vi "PH_PPPA_PowerUnit.PC_StateDumpRoss.vi"(0 "i ref in":refnum<vi>, 3 "Dump Ross State":T1 items=["no info", "off/false/out", "on/true/in", "Failure", "Alarm", "Status 1", "Status 2", "Status 3"], 4 "not linked":bool, 5 "error in (no error)":errorcluster) -> (14 "i ref out":refnum<vi>, 19 "error out":errorcluster)   [LabVIEW 2014, in "PH_PPPA_PowerUnit.lvlib"]
doc: "This VI writes the Dump Ross Relais Tag values to own attributes, calculates the state of the device and sets the GUI object."
uses:
  PH_PPPA_PowerUnit.lvlib
  PH_StatusHandler/PH_StatusHandler.Status.ctl
  PH_Common/PH_Common.lvlib
  PH_StatusHandler/PH_StatusHandler.lvlib
  PH_Beckhoff_PP_PU/PH_Beckhoff_PP_PU.lvlib
  PH_PowerUnit_BaseClass/PH_PowerUnit_BaseClass.lvlib
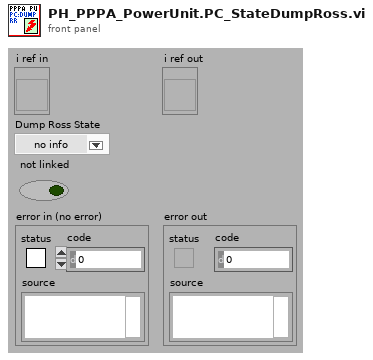
[diagram p1: front panel]
types:
  T1 = typedef "PH_StatusHandler.lvlib/PH_StatusHandler.Status.ctl" = i16
  T2 = typedef "PH_PowerUnit_BaseClass.lvlib/PH_PowerUnit_BaseClass.i attribute.ctl" = cluster{"Constructor finished":bool, "PU":cluster{"In use":bool, "Service ID in use":i32, "GUI Ref":refnum<vi>}, "Enabling":cluster{"State":T3, "GUI Ref":refnum<vi>}, "Timing":cluster{"Last Shot":dbl, "Time between Shots [Sec]":dbl, "Waiting Time over?":bool, "Service ID Waiting Time":i32, "GUI Ref":refnum<vi>, "Instance":cluster{"Status":T1, "linked?":bool, "GUI Ref":refnum<vi>}}, "Sequencer":cluster{"SM State":string, "GUI Ref":refnum<vi>, "linked":bool}, "Subscribed Trendmssgs":cluster{"Tagname":string, "Status":T1, "linked?":bool, "Shot Condition":T1, "GUI Ref":refnum<vi>}[], "PP PU":T4, "Default Voltage (V)":dbl, "GUI Refs":T5, "PSDB data":cluster{"Shot Voltage [V]":dbl, "State TO SM":T6, "Write 2 early":bool}, "State TO SM":T6}
  T3 = typedef "PH_SystemInformation.lvlib/PH_SystemInformationEnabling State.ctl" = i32
  T4 = typedef "PH_PP_Common.lvlib/PH_PP_Common.PUs.ctl" = enum16{"no Info", "PA-19mm-1", "PA-19mm-2", "PA-45mm-PILC", "PA-45mm-MAIN", "MA-PU-1", "MA-PU-2", "MA-PU-3", "MA-PU-4", "MA-PU-5", "MA-PU-6", "MA-FR", "MA-PILC", "PA-45mm-DP"}
  T5 = typedef "PH_PowerUnit_BaseClass.lvlib/PH_PowerUnit_BaseClass.GUI Refs.ctl" = cluster{"Delete Inst":refnum<vi>, "State TO SM":refnum<vi>, "State SM":refnum<vi>, "Fire":refnum<vi>}
  T6 = typedef "PH_PowerUnit_BaseClass.lvlib/PH_PowerUnit_BaseClass.SM States.ctl" = enum16{".", "Stand by", "Switch PU on", "Configure", "Set Default Voltage", "Set STANDBY", "Set READY", "Wait for Shot Cmd", "Open Dump Rods", "Open Ross Relais", "Close Ross Relais", "Switch PSU on", "Switch PSU off", "Charge", "Switch GD Channel on", "Close Dump Rods", "Rods-TO", "RR-TO", "PSU-TO", "Trigger-TO"}
  T7 = typedef "PH_PPPA_PowerUnit.lvlib/PH_PPPA_PowerUnit.i attribute.ctl" = cluster{"GUI Refs":cluster{"Ignitron":refnum<vi>, "Rossrelais":refnum<vi>, "Set Voltage":refnum<vi>, "PSU":refnum<vi>, "EOC":refnum<vi>, "Trigger":refnum<vi>}, "Ignitron":T8, "PSU":T9, "Dump Ross Relais":T10, "Trigger":cluster{"State Device":T1, "linked?":bool}, "Timing Settings":cluster{"Prdc Fast?":bool, "Default Value Periodic Interval":i32, "Mercury on since":dbl, "Warm up Time Mercury [s]":dbl}, "Set Voltage [V]":dbl, "19er Ignitionbox":string}
  T8 = typedef "PH_PP_Common.lvlib/PH_PP_Common.Ignitron Attributes.ctl" = cluster{"State Device":T1, "linked?":bool}
  T9 = typedef "PH_PP_Common.lvlib/PH_PP_Common.PSU Attributes.ctl" = cluster{"lower limit [V]":dbl, "upper limit [V]":dbl, "Voltage set":bool, "State Device":T1, "linked?":bool}
  T10 = typedef "PH_PP_Common.lvlib/PH_PP_Common.Ross Relais Attributes.ctl" = cluster{"State Device":T1, "linked?":bool}
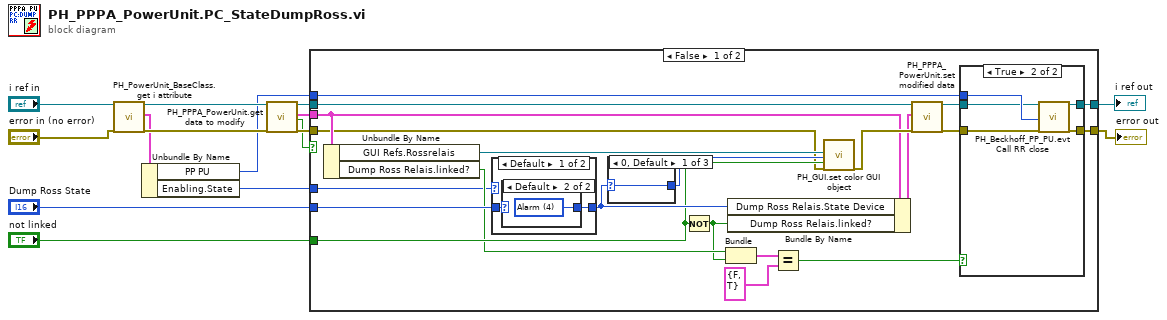
[diagram p0: block diagram]
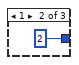
[diagram p3: hidden frame]
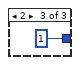
[diagram p4: hidden frame]
diagram:
  n1 = call "PH_PowerUnit_BaseClass.get i attribute.vi"("i ref in"="i ref in", "error in (no error)"="error in (no error)") -> ("i ref out"=w4:refnum<vi>, "i attribute"=w3:T2, "error out"=w6:errorcluster)  [unwired: 15 in]
  n2 = Unbundle By Name(w3) -> ("PP PU"=w1:T4, "Enabling.State"=w2:T3)
  n3 = call "PH_PPPA_PowerUnit.get data to modify.vi"("i ref in"=w4, "error in (no error)"=w6) -> ("i ref out"=w15:refnum<vi>, "i attribute"=w13:T7, "timed out"=w12:bool, "error out"=w14:errorcluster)  [unwired: 14 in]
  n4 = case shown="False" w12 {
    tunnel: w15 -> [w19 w53]
    tunnel: [w23 w53] -> w11
    tunnel: w14 -> [w18 w52]
    tunnel: [w21 w52] -> w10
    tunnel: w13 -> [w33 _]
    tunnel: "Dump Ross State" -> [w32 _]
    tunnel: "not linked" -> [w29 _]
    tunnel: w2 -> [w17 _]
    tunnel: w1 -> [w16 _]
    frame False {
      n5 = Unbundle By Name(w33) -> ("GUI Refs.Rossrelais"=w34:refnum<vi>, "Dump Ross Relais.linked?"=w28:bool)
      n6 = case shown="Default" w17 {
        tunnel: w32 -> [w48 w51]
        tunnel: [w47 w51] -> w31
        frame Default {
          n7 = case shown="Default" w48 {
            selector: w48 -> [w49 _]
            tunnel: [w49 w50] -> w47
            frame 2 {
            }
            frame Default {
              w50 = T1 4 items=["no info", "off/false/out", "on/true/in", "Failure", "Alarm", "Status 1", "Status 2", "Status 3"] ("Dump Ross State")
            }
          }
        }
        frame 1 {
        }
      }
      n8 = case shown="0, Default" w31 {
        selector: w31 -> [w44 _ _]
        tunnel: [w44 2 ("State") 1 ("State")] -> w30
        frame 0, Default {
        }
        frame 1 {
        }
        frame 2 {
        }
      }
      n9 = Not(x=w29) -> (.not. x?=w27:bool)
      n10 = Bundle("linked?"=w28, w27) -> (w26:cluster{"linked?":bool, bool})  [unwired: 1 in]
      n11 = Bundle By Name(cluster=w33, "Dump Ross Relais.State Device"=w31, "Dump Ross Relais.linked?"=w27) -> (w35:T7)
      n12 = Equal?(x=w26, y=cluster{"linked?":bool, bool} {"linked?"=FALSE, TRUE}) -> (x = y?=w20:bool)
      n13 = call "PH_GUI.set color GUI object.vi"("GUI object Ref"=w34, "State"=w30, "Blinking? (false)"=w29, "error in (no error)"=w18) -> ("error out"=w36:errorcluster)  [unwired: 15 in]
      n14 = call "PH_PPPA_PowerUnit.set modified data.vi"("i ref in"=w19, "i attribute"=w35, "error in (no error)"=w36) -> ("i ref out"=w24:refnum<vi>, "error out"=w22:errorcluster)  [unwired: 15 in]
      n15 = case shown="True" w20 {
        tunnel: w24 -> [w38 w39]
        tunnel: [w38 w43] -> w23
        tunnel: w22 -> [w37 w40]
        tunnel: [w37 w42] -> w21
        tunnel: w16 -> [_ w41]
        frame False {
        }
        frame True {
          n16 = call "PH_Beckhoff_PP_PU.evt Call RR close.vi"("i ref in"=w39, "PU"=w41, "error in"=w40) -> ("i ref out"=w43:refnum<vi>, "error out"=w42:errorcluster)  [unwired: 15 in]
        }
      }
    }
    frame True {
    }
  }
  "error out" <- w10
  "i ref out" <- w11
